vi "CelsiusToFar.vi"() -> ()   [LabVIEW 2019]
panel:
  out "Far":dbl(slide) scale=0.0..150.0
  in  "Celsius":dbl(slide) scale=0.0..100.0
  out "TempInFar":dbl
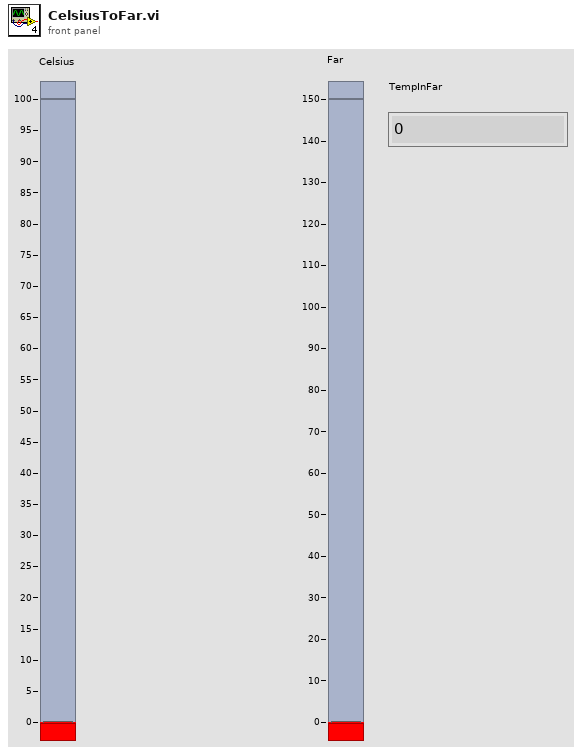
[diagram p1: front panel]
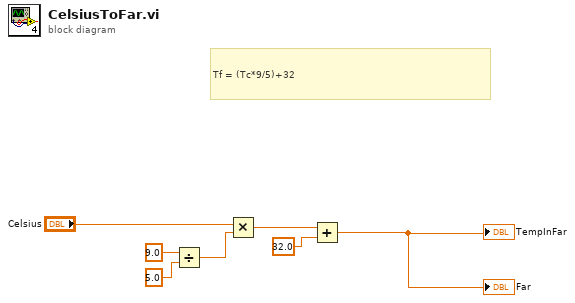
[diagram p0: block diagram]
diagram:
  # "Tf = (Tc*9/5)+32"
  n1 = Divide(x=9.0, y=5.0 ("x")) -> (x/y=w5:dbl)
  n2 = Multiply(x="Celsius", y=w5) -> (x*y=w4:dbl)
  n3 = Add(x=w4, y=32.0 ("x")) -> (x+y=→"TempInFar" →"Far":dbl)
